vi "Camera indicator mapping.vi"(9 "Dynamic image update params in":T1, 10 "Selected imaging view name":string="C2", 11 "Selected label name":string="Image label 1") -> (3 "Dynamic image update params out":T1)   [LabVIEW 2019, in "ZenGage v3.0 UI.lvclass"]
uses:
  ZenGage v3.0 UI.lvclass
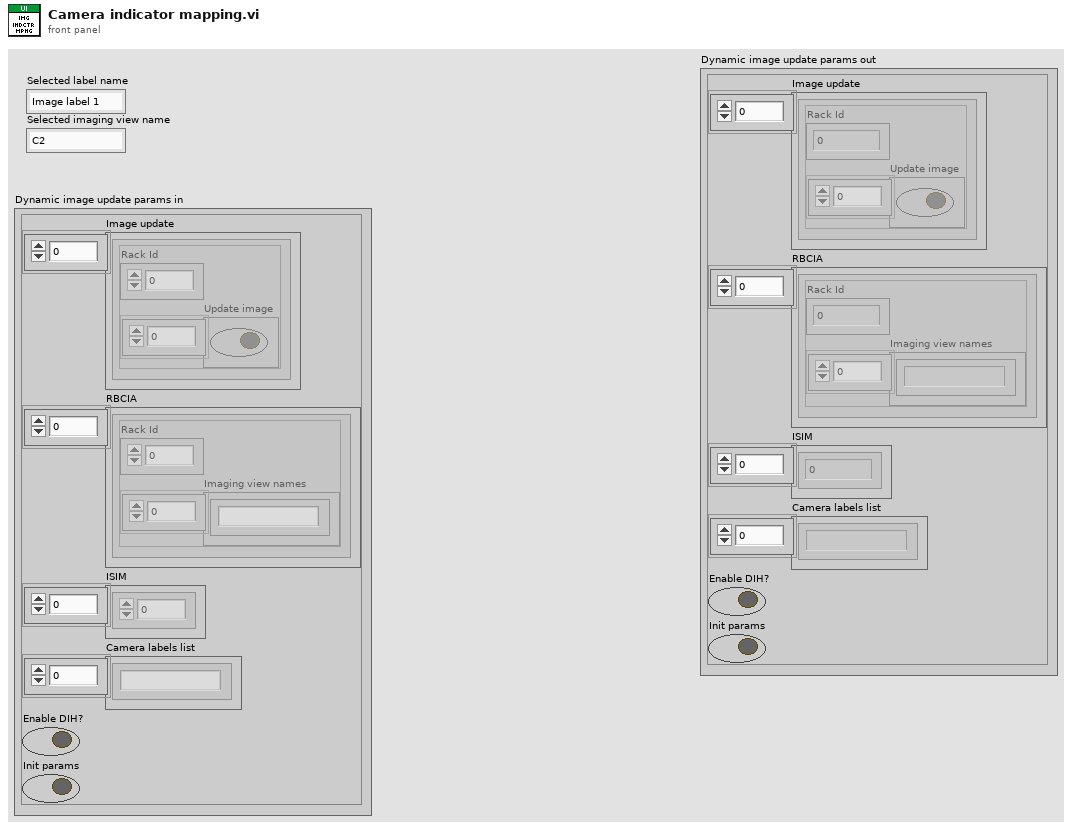
[diagram p1: front panel]
types:
  T1 = cluster{"Image update":cluster{"Rack Id":i32, "Update image":bool[]}[], "RBCIA":cluster{"Rack Id":u8, "Imaging view names":string[]}[], "ISIM":u8[], "Camera labels list":string[], "Enable DIH?":bool, "Init params":bool}
  T2 = cluster{"Rack Id":u8, "Imaging view names":string[]}[]
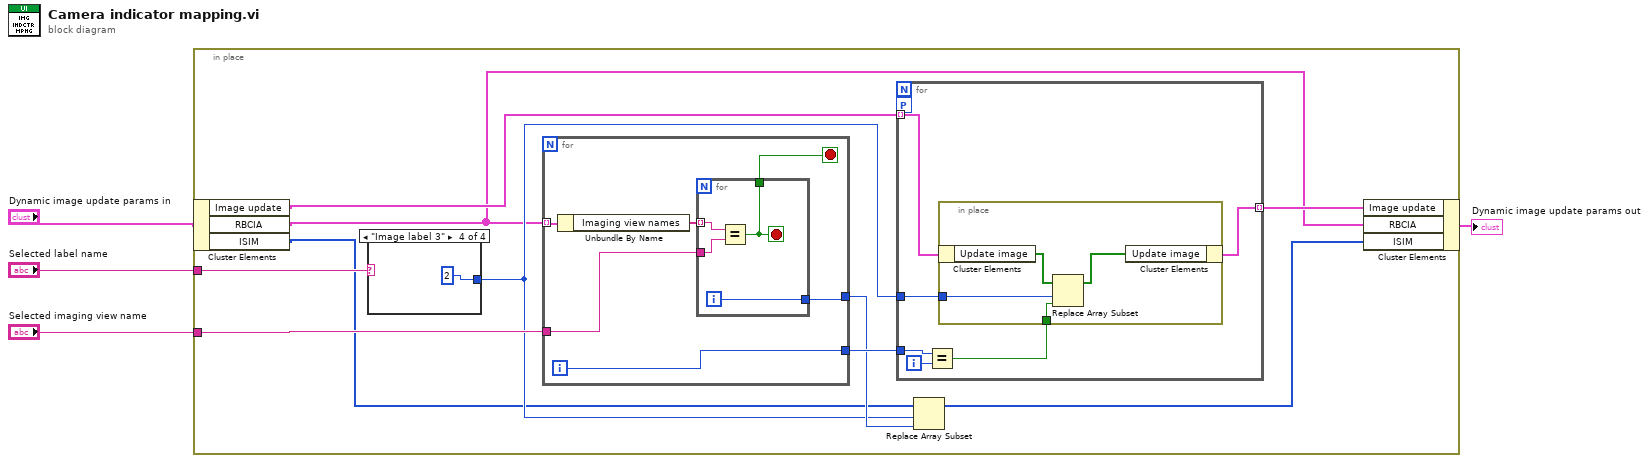
[diagram p0: block diagram]
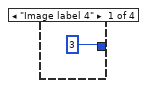
[diagram p2: hidden frame]
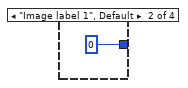
[diagram p3: hidden frame]
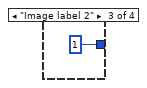
[diagram p4: hidden frame]
diagram:
  n1 = in-place {
    in-place-border: "Selected label name" -> [w14]
    in-place-border: "Selected imaging view name" -> [w13]
    n2 = in-place-cluster #1("Dynamic image update params in") -> ("Image update"=w9:cluster{"Rack Id":i32, "Update image":bool[]}[], "RBCIA"=w5:T2, "ISIM"=w8:u8[])
    n3 = case shown="\"Image label 3\"" w14 {
      tunnel: [3 0 1 2] -> w10
      frame "Image label 4" {
      }
      frame "Image label 1", Default {
      }
      frame "Image label 2" {
      }
      frame "Image label 3" {
      }
    }
    n4 = for {
      tunnel: w5 -> [w30] mode=indexing
      tunnel: w13 -> [w28]
      tunnel: [w27] -> w12
      tunnel: [w26] -> w11
      i -> [w27]
      stop <- w25 stop-if-true
      n5 = Unbundle By Name(w30) -> ("Imaging view names"=w29:string[])
      n6 = for {
        tunnel: w29 -> [w34] mode=indexing
        tunnel: w28 -> [w33]
        tunnel: [w32] -> w26
        tunnel: [w31] -> w25
        i -> [w32]
        stop <- w31 stop-if-true
        n7 = Equal?(x=w34, y=w33) -> (x = y?=w31:bool)
      }
    }
    n8 = for {
      tunnel: w9 -> [w16] mode=indexing
      tunnel: w12 -> [w19]
      tunnel: w10 -> [w18]
      tunnel: [w15] -> w7 mode=indexing
      workers-P: _ -> [_]
      i -> [w20]
      n9 = Equal?(x=w19, y=w20) -> (x = y?=w17:bool)
      n10 = in-place {
        in-place-border: w18 -> [w24]
        in-place-border: w17 -> [w23]
        n11 = in-place-cluster #2(w16) -> ("Update image"=w22:bool[])
        n12 = Replace Array Subset(array=w22, new element=w23, index=w24) -> (w21:bool[])
        n13 = in-place-cluster #2("Update image"=w21) -> (w15:cluster{"Rack Id":i32, "Update image":bool[]})
      }
    }
    n14 = Replace Array Subset(array=w8, new element=w11, index=w10) -> (w6:u8[])
    n15 = in-place-cluster #1("Image update"=w7, "RBCIA"=w5, "ISIM"=w6) -> (→"Dynamic image update params out":T1)
  }
